vi "CAL_LOAD_L.vi"(0 "Param In":T2, 1 "Force":sgl[](array[numeric]), 2 "Control param In":T1={"L_velocity"=10000, "L_Power"=0.0, "R_velocity"=10000, "R_Power"=0.0, "T_param_L"={"Onset start"=0.0, "Onset end"=5.0, "Peak start"=10.0, "Release start"=60.0, "slang"=80.0, "Peak end"=58.0}, "T_param_R"={"Onset start"=0.0, "Onset end"=5.0, "Peak start"=10.0, "Release start"=60.0, "slang"=80.0, "Peak end"=58.0}, "Initialize?"=FALSE, "CAN read?"=FALSE, "Optimal count"=0}, 3 "에러 입력(에러 없음) 2":errorcluster caption="에러 입력(에러 없음)") -> (4 "Load_Onset":sgl, 5 "Load_Peak":sgl, 7 "Param Out":T2, 10 "에러 입력(에러 없음) 3":errorcluster caption="에러 입력(에러 없음)")   [LabVIEW 2019]
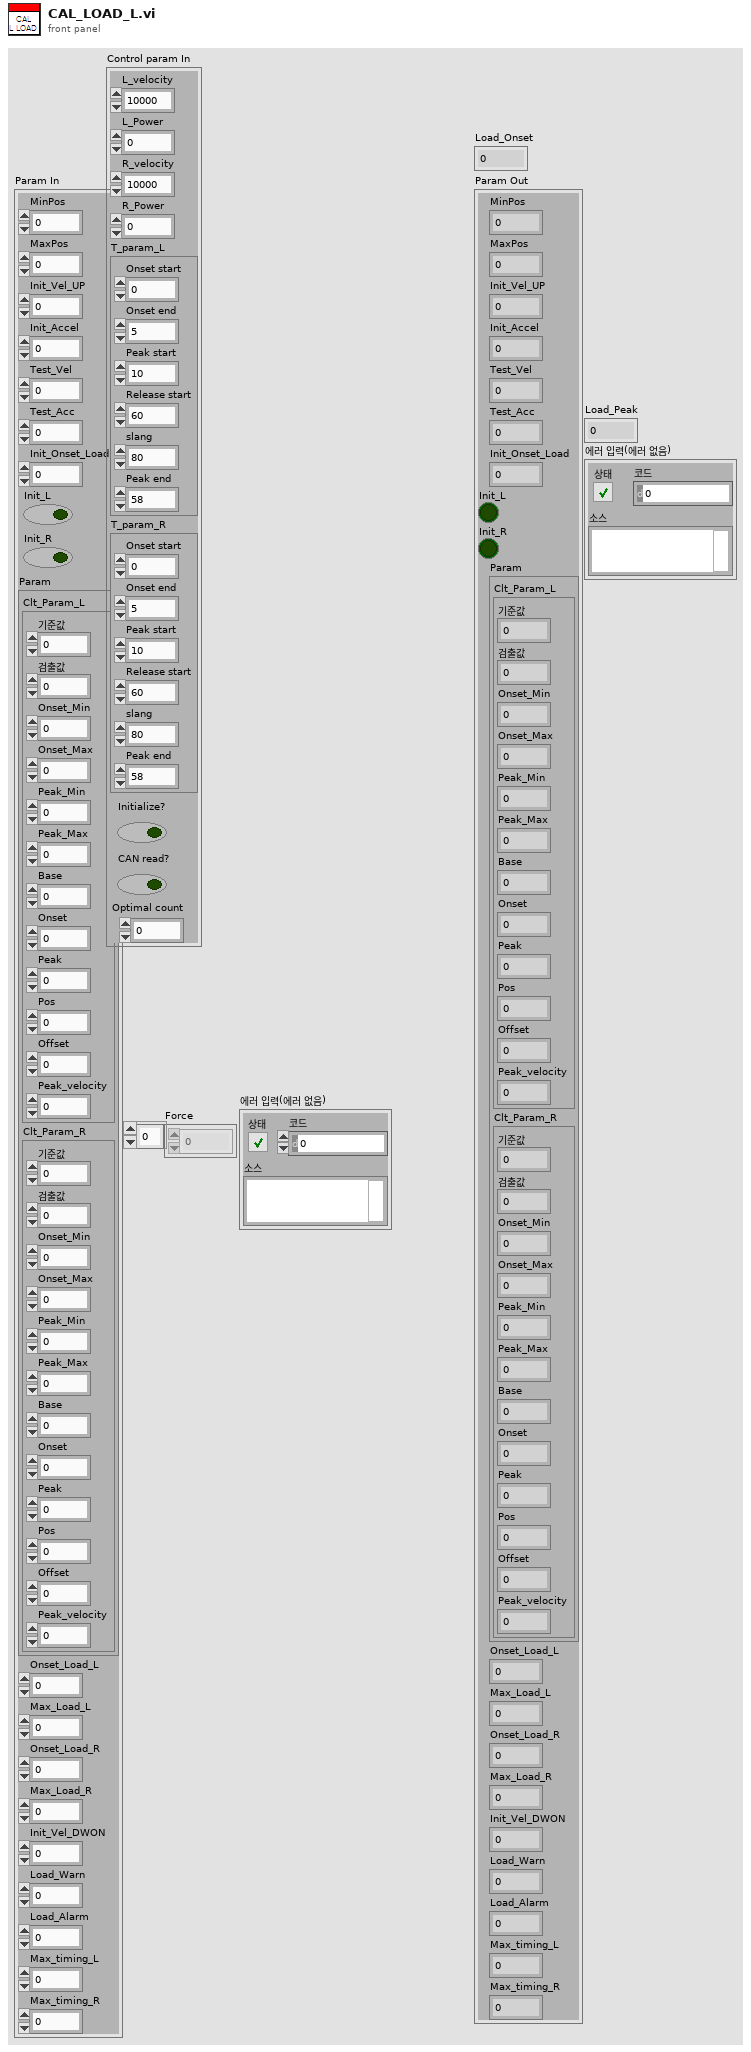
[diagram p1: front panel]
types:
  T1 = cluster{"L_velocity":u32, "L_Power":sgl, "R_velocity":u32, "R_Power":sgl, "T_param_L":cluster{"Onset start":sgl, "Onset end":sgl, "Peak start":sgl, "Release start":sgl, "slang":sgl, "Peak end":sgl}, "T_param_R":cluster{"Onset start":sgl, "Onset end":sgl, "Peak start":sgl, "Release start":sgl, "slang":sgl, "Peak end":sgl}, "Initialize?":bool, "CAN read?":bool, "Optimal count":i32}
  T2 = cluster{"MinPos":i32, "MaxPos":i32, "Init_Vel_UP":i32, "Init_Accel":u32, "Test_Vel":i32, "Test_Acc":u32, "Init_Onset_Load":sgl, "Init_L":bool, "Init_R":bool, "Param":cluster{"Clt_Param_L":cluster{"기준값":sgl, "검출값":sgl, "Onset_Min":sgl, "Onset_Max":sgl, "Peak_Min":sgl, "Peak_Max":sgl, "Base":i32, "Onset":i32, "Peak":i32, "Pos":i32, "Offset":sgl, "Peak_velocity":i32}, "Clt_Param_R":cluster{"기준값":sgl, "검출값":sgl, "Onset_Min":sgl, "Onset_Max":sgl, "Peak_Min":sgl, "Peak_Max":sgl, "Base":i32, "Onset":i32, "Peak":i32, "Pos":i32, "Offset":sgl, "Peak_velocity":i32}}, "Onset_Load_L":sgl, "Max_Load_L":sgl, "Onset_Load_R":sgl, "Max_Load_R":sgl, "Init_Vel_DWON":i32, "Load_Warn":sgl, "Load_Alarm":sgl, "Max_timing_L":sgl, "Max_timing_R":sgl}
  T3 = cluster{"Onset start":sgl, "Onset end":sgl, "Peak start":sgl, "Release start":sgl, "slang":sgl, "Peak end":sgl}
  T4 = cluster{"Onset start":i32, "Onset end":i32, "Peak start":i32, "Release start":i32, "slang":i32, "Peak end":i32}
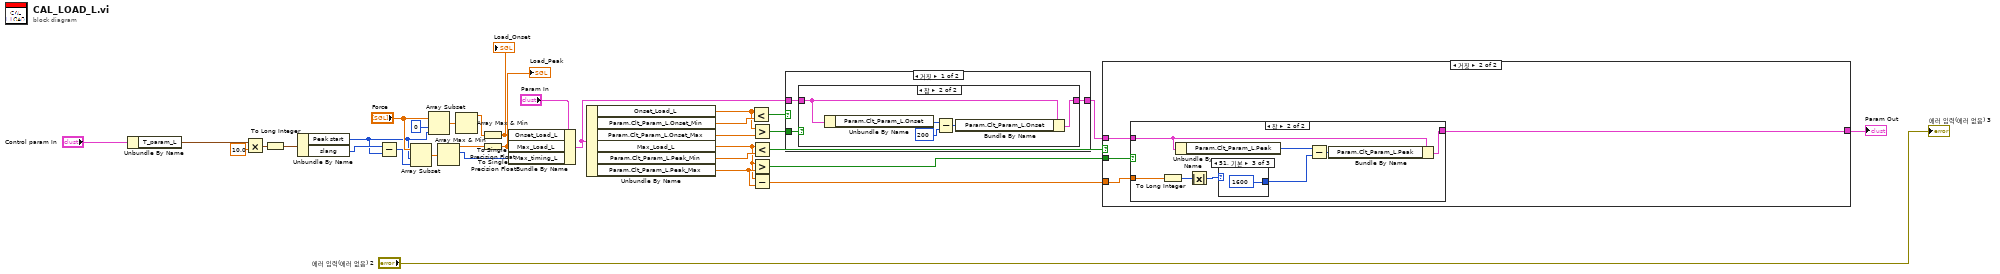
[diagram p0: block diagram]
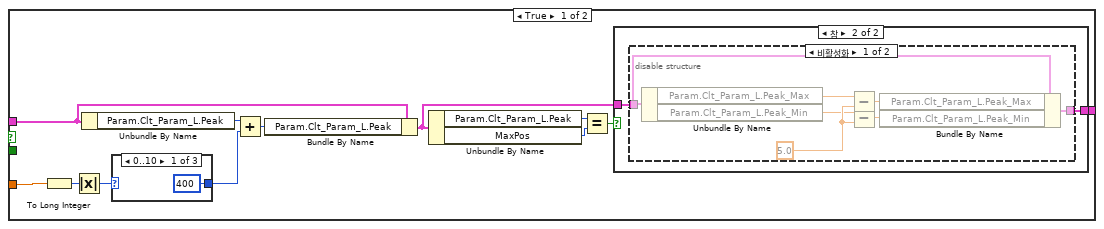
[diagram p2: hidden frame]
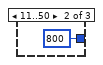
[diagram p5: hidden frame]
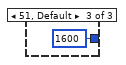
[diagram p6: hidden frame]
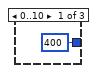
[diagram p8: hidden frame]
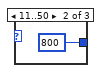
[diagram p9: hidden frame]
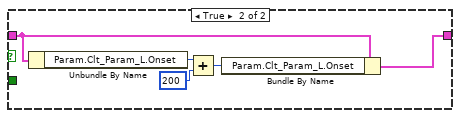
[diagram p11: hidden frame]
diagram:
  n1 = Unbundle By Name("Control param In") -> ("T_param_L"=w5:T3)
  n2 = Multiply(x=w5, y=sgl 10.0) -> (x*y=w15:T3)
  n3 = To Long Integer(number=w15) -> (32bit integer=w7:T4)
  n4 = Unbundle By Name(w7) -> ("Peak start"=w9:i32, "slang"=w14:i32)
  n5 = Subtract(x=w14, y=w9) -> (x-y=w8:i32)
  n6 = Array Subset(array="Force", index=w9, length=w8) -> (w22:sgl[])
  n7 = Array Subset(array="Force", index=0 ("인덱스"), length=w9) -> (w23:sgl[])
  n8 = Array Max & Min(array=w22) -> (max value=w20:sgl, max index (indices)=w17:i32)  [unwired: 2 out]
  n9 = Array Max & Min(array=w23) -> (max value=w12:sgl)  [unwired: 3 out]
  n10 = To Single Precision Float(number=w12) -> (single precision float=w18:sgl)
  "Load_Onset" <- w18
  n11 = To Single Precision Float(number=w20) -> (single precision float=w19:sgl)
  "Load_Peak" <- w19
  n12 = Bundle By Name(cluster="Param In", "Onset_Load_L"=w18, "Max_Load_L"=w19, "Max_timing_L"=w17) -> (w10:T2)
  n13 = Unbundle By Name(w10) -> ("Onset_Load_L"=w31:sgl, "Param.Clt_Param_L.Onset_Min"=w33:sgl, "Param.Clt_Param_L.Onset_Max"=w32:sgl, "Max_Load_L"=w1:sgl, "Param.Clt_Param_L.Peak_Min"=w30:sgl, "Param.Clt_Param_L.Peak_Max"=w24:sgl)
  n14 = Less?(x=w31, y=w33) -> (x < y?=w29:bool)
  n15 = Greater?(x=w31, y=w32) -> (0:w28:bool)
  n16 = Less?(x=w1, y=w30) -> (x < y?=w27:bool)
  n17 = Greater?(x=w1, y=w24) -> (0:w26:bool)
  n18 = Subtract(x=w1, y=w24) -> (x-y=w2:sgl)
  n19 = case shown="거짓" w29 {
    tunnel: w10 -> [w36 w44]
    tunnel: w28 -> [w34 _]
    tunnel: [w35 w43] -> w25
    frame False {
      n20 = case shown="참" w34 {
        tunnel: w36 -> [w37 w40]
        tunnel: [w37 w38] -> w35
        frame False {
        }
        frame True {
          n21 = Unbundle By Name(w40) -> ("Param.Clt_Param_L.Onset"=w42:i32)
          n22 = Subtract(x=w42, y=200) -> (x-y=w39:i32)
          n23 = Bundle By Name(cluster=w40, "Param.Clt_Param_L.Onset"=w39) -> (w38:T2)
        }
      }
    }
    frame True {
      n24 = Unbundle By Name(w44) -> ("Param.Clt_Param_L.Onset"=w47:i32)
      n25 = Add(x=w47, y=200) -> (x+y=w45:i32)
      n26 = Bundle By Name(cluster=w44, "Param.Clt_Param_L.Onset"=w45) -> (w43:T2)
    }
  }
  n27 = case shown="거짓" w27 {
    tunnel: w25 -> [w54 w77]
    tunnel: [w53 w76] -> w6
    tunnel: w26 -> [_ w75]
    tunnel: w2 -> [w48 w74]
    frame True {
      n28 = To Long Integer(number=w48) -> (32bit integer=w49:i32)
      n29 = Absolute Value(x=w49) -> (abs(x)=w50:i32)
      n30 = Unbundle By Name(w54) -> ("Param.Clt_Param_L.Peak"=w59:i32)
      n31 = case shown="0..10" w50 {
        tunnel: [400 ("y") 800 ("y") 1600 ("y")] -> w57
        frame 0..10 {
        }
        frame 11..50 {
        }
        frame 51, Default {
        }
      }
      n32 = Add(x=w59, y=w57) -> (x+y=w58:i32)
      n33 = Bundle By Name(cluster=w54, "Param.Clt_Param_L.Peak"=w58) -> (w52:T2)
      n34 = Unbundle By Name(w52) -> ("Param.Clt_Param_L.Peak"=w56:i32, "MaxPos"=w51:i32)
      n35 = Equal?(x=w56, y=w51) -> (x = y?=w55:bool)
      n36 = case shown="참" w55 {
        tunnel: w52 -> [w60 w62]
        tunnel: [w60 w61] -> w53
        frame False {
        }
        frame True {
          n37 = disable-structure shown="비활성화" {
            disable-tunnel: w62 -> [w66 w70]
            disable-tunnel: [w63 w70] -> w61
            frame Disabled {
              w69 = sgl 5.0
              n38 = Unbundle By Name(w66) -> ("Param.Clt_Param_L.Peak_Max"=w68:sgl, "Param.Clt_Param_L.Peak_Min"=w64:sgl)
              n39 = Subtract(x=w68, y=w69) -> (x-y=w67:sgl)
              n40 = Subtract(x=w64, y=w69) -> (x-y=w65:sgl)
              n41 = Bundle By Name(cluster=w66, "Param.Clt_Param_L.Peak_Max"=w67, "Param.Clt_Param_L.Peak_Min"=w65) -> (w63:T2)
            }
            frame Enabled {
            }
          }
        }
      }
    }
    frame False {
      n42 = case shown="참" w75 {
        tunnel: w77 -> [w78 w85]
        tunnel: [w78 w83] -> w76
        tunnel: w74 -> [_ w79]
        frame False {
        }
        frame True {
          n43 = To Long Integer(number=w79) -> (32bit integer=w82:i32)
          n44 = Unbundle By Name(w85) -> ("Param.Clt_Param_L.Peak"=w86:i32)
          n45 = Absolute Value(x=w82) -> (abs(x)=w81:i32)
          n46 = case shown="51, 기본" w81 {
            tunnel: [400 ("y") 800 ("y") 1600 ("y")] -> w80
            frame 0..10 {
            }
            frame 11..50 {
            }
            frame 51, Default {
            }
          }
          n47 = Subtract(x=w86, y=w80) -> (x-y=w84:i32)
          n48 = Bundle By Name(cluster=w85, "Param.Clt_Param_L.Peak"=w84) -> (w83:T2)
        }
      }
    }
  }
  "Param Out" <- w6
  "에러 입력(에러 없음) 3" <- "에러 입력(에러 없음) 2"
